vi "Assert Valid Refnum.vi"(4 "Execution time (s)":dbl=-1.0, 5 "Assert Only? (F)":bool, 6 "error code (1)":i32=1, 7 "Label (\"\")":string, 8 "error in (no error)":errorcluster, 9 "Register with caller test (F)":bool, 11 "Refnum":variant) -> (0 "error out":errorcluster, 2 "Properties.Assert":refnum<class "Properties.Assert.lvclass">)   [LabVIEW 2013, in "Caraya.lvlib" / "Assert.lvclass"]
doc: "Asserts that a <B>refnum</B> is valid."
uses:
  Assert.lvclass
  Properties.Assert/Properties.Assert.lvclass
  Properties/Properties.lvclass
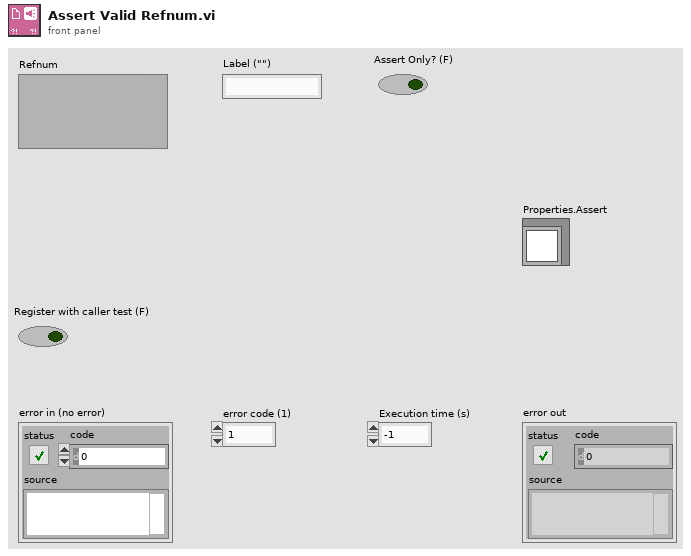
[diagram p1: front panel]
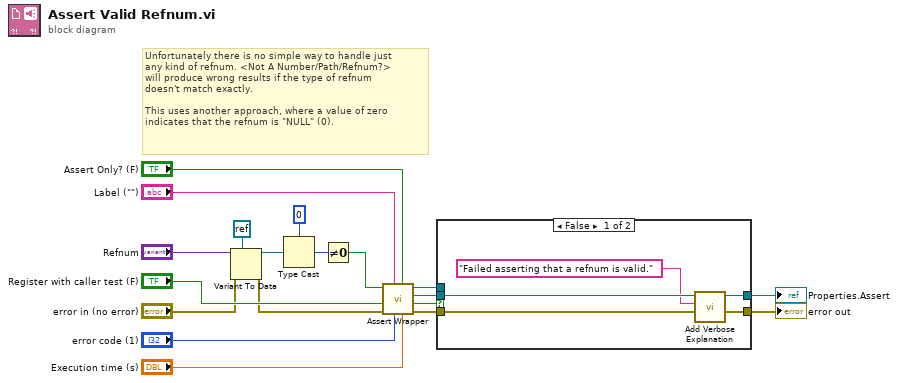
[diagram p0: block diagram]
diagram:
  # "Unfortunately there is no simple way to handle just\nany kind of refnum. <Not A Number/Path/Refnum?>\nwill produce wrong results if the type of refnum\ndoesn't match exactly.\n\nThis uses another approach, where a value of zero\nindicates that the refnum is \"NULL\" (0)."
  n1 = Variant To Data(error in="error in (no error)", type=refnum<k0> refnum, Variant="Refnum") -> (data=w4:refnum<k0>, error out=w6:errorcluster)
  n2 = Type Cast(type=u64 0, x=w4) -> (*(type *) &x=w2:u64)
  n3 = Not Equal To 0?(x=w2) -> (x != 0?=w1:bool)
  n4 = call "Assert Wrapper.vi"("Execution time (s)"="Execution time (s)", "Assert Only? (F)"="Assert Only? (F)", "error code (1)"="error code (1)", "Label"="Label (\"\")", "error in (no error)"=w6, "Register with caller test (F)"="Register with caller test (F)", "Assert?"=w1) -> ("error out"=w10:errorcluster, "Verbose"=w14:bool, "Properties.Assert"=w12:refnum<class "Properties.Assert.lvclass">, "Assert out"=w13:refnum<class "Assert.lvclass">)  [unwired: 1 in]
  n5 = case shown="False" w14 {
    tunnel: w13 -> [_ _]
    tunnel: w12 -> [w22 w26]
    tunnel: [w23 w25] -> w11
    tunnel: w10 -> [w24 w25]
    tunnel: [w21 w26] -> w9
    frame False {
      n6 = call "Add Verbose Explanation.vi"("error in (no error)"=w24, "Verbose Explanation"="Failed asserting that a refnum is valid.", "Properties"=w22) -> ("error out"=w23:errorcluster, "Properties"=w21:refnum<class "Properties.Assert.lvclass">)  [unwired: 7 in]
    }
    frame True {
    }
  }
  "error out" <- w11
  "Properties.Assert" <- w9
